vi "Practica 13 - subVoltaje.vi"(1 "RT":dbl, 2 "E":dbl, 3 "Rx":dbl) -> (0 "Vx":dbl)   [LabVIEW 2023]
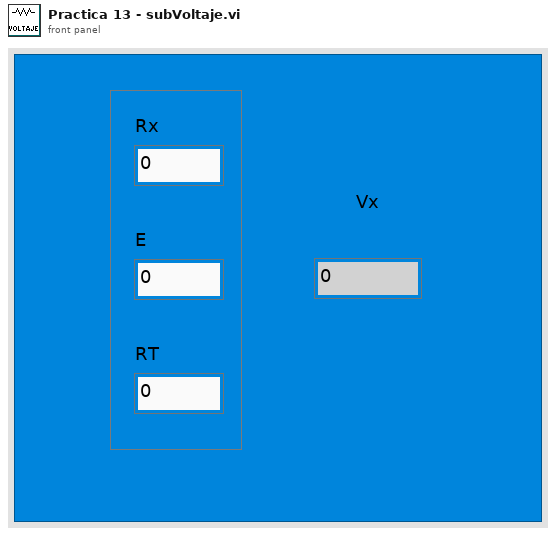
[diagram p1: front panel]
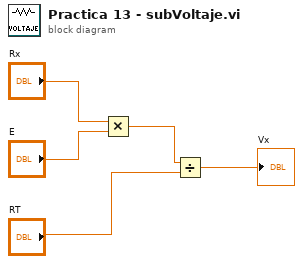
[diagram p0: block diagram]
diagram:
  n1 = Multiply(x="Rx", y="E") -> (x*y=w3:dbl)
  n2 = Divide(x=w3, y="RT") -> (x/y=→"Vx":dbl)
